vi "Setup.vi"(0 "Power Supply VISA resource name":refnum<visa-resource-name>, 1 "Set Voltage":dbl=3.3 format="%#_13g", 2 "ADC Input Channel 2":tag="cDAQ2Mod3/ai0", 3 "ADC Sample Mode":i32(ring)=10123 items=["Finite Samples"=10178, "Continuous Samples"=10123, "Hardware Timed Single Point"=12522], 4 "Set Max Current for FP":dbl=0.25 format="%#_13g", 5 "Sample Length for ADC mean":i32=100, 6 "ADC Minimum Value":dbl=-10.0 format="%0.2f", 7 "ADC Sampling Rate":dbl=10000.0 format="%0.2f", 8 "ADC Maximum Value":dbl=10.0 format="%0.2f") -> (12 "Sample Length for ADC mean 2":i32=100, 13 "Beginning Time Stamp":timestamp, 14 "DAQ Task Out":refnum<k21>, 15 "DAQ Error Out":errorcluster, 16 "VISA resource name out":refnum<visa-resource-name>, 17 "Power Supply Error Out":errorcluster, 18 "LINX Resource":T1={"IO"=enum."Remote", "Interface"=enum."Serial", "LINX Device Config"={"Interface"=enum."Serial", "COM Port"="COM13", "TCP Configuration"={"IP Address"="", "Port"=0}, "Device Family"=1, "Device ID"=1, "Device Name"="myRIO-1900", "TCP Ref"=refnum, "Channels"={"DI"=[0, 1, 2, 3, 4, 5, 6, 7, 8, 9, 10, 11, 12, 13, 14, 15, 16, 17, 18, 19, 20, 21, 22, 23, 24, 25, 26, 27, 28, 29, 30, 31, 32, 33, 34, 35, 36, 37, 38, 39, 40, 41, 42, 43, 44, 45, 46], "DO"=[0, 1, 2, 3, 4, 5, 6, 7, 8, 9, 10, 11, 12, 13, 14, 15, 16, 17, 18, 19, 20, 21, 22, 23, 24, 25, 26, 27, 28, 29, 30, 31, 32, 33, 34, 35, 36, 37, 38, 39, 40, 41, 42, 43, 44, 45, 46], "AI"=[0, 1, 2, 3, 4, 5, 6, 7, 8, 9, 10, 11], "AO"=[], "PWM"=[3, 5, 6, 9, 10], "QE"=[], "UART"=[0, 1], "I2C 2"=[0], "SPI"=[0], "CAN"=[], "Servo"=[], "AI Ref (V)"=0.0, "AI Resolution (Bits)"=0, "AO Ref (V)"=0.0, "AO Resolution (Bits)"=0}}}, 19 "Arduino Error Out":errorcluster={"status"=FALSE, "code"=1073676294, "source"="VISA Read in LVH-LINX.lvlib:Device.lvlib:Serial Read.vi->LVH-LINX.lvlib:Device.lvlib:Wait For Packet.vi->LVH-LINX.lvlib:Device.lvlib:Send Command.vi->LVH-LINX.lvlib:Device.lvlib:Get DIO Channels.vi->LVH-LINX.lvlib:Device.lvlib:Load Device Config.vi->LVH-LINX.lvlib:Device.lvlib:Initialize Device.vi->LVH-LINX.lvlib:Initialize.vi->Untitled 2"})   [LabVIEW 2018]
uses:
  <vilib>/MakerHub/LINX/Private/Type Defs/LINX Ref.ctl
  <vilib>/MakerHub/LINX/Private/Type Defs/Platform.ctl
  <vilib>/MakerHub/LINX/Private/Type Defs/Interface.ctl
  <vilib>/MakerHub/LINX/Private/Device/Type Defs/LINX Device Config.ctl
  <vilib>/MakerHub/LINX/Private/Device/Type Defs/TCP Config.ctl
  <vilib>/MakerHub/LINX/Private/Device/Type Defs/Channels.ctl
  <vilib>/MakerHub/LINX/Public/Utilities/Open Serial.vi
  <vilib>/DAQmx/create/channels.llb/DAQmx Create Channel (AI-Voltage-Basic).vi
  <vilib>/DAQmx/configure/timing.llb/DAQmx Timing (Sample Clock).vi
  <instrlib>/XP Power PLS600/XP Power PLS600.lvlib
  <vilib>/MakerHub/LINX/LMH-LINX.lvlib
  <vilib>/MakerHub/LINX/Private/Device/Device.lvlib
panel:
  in  "Serial Port for Arduino":refnum<visa-resource-name>="N/A"
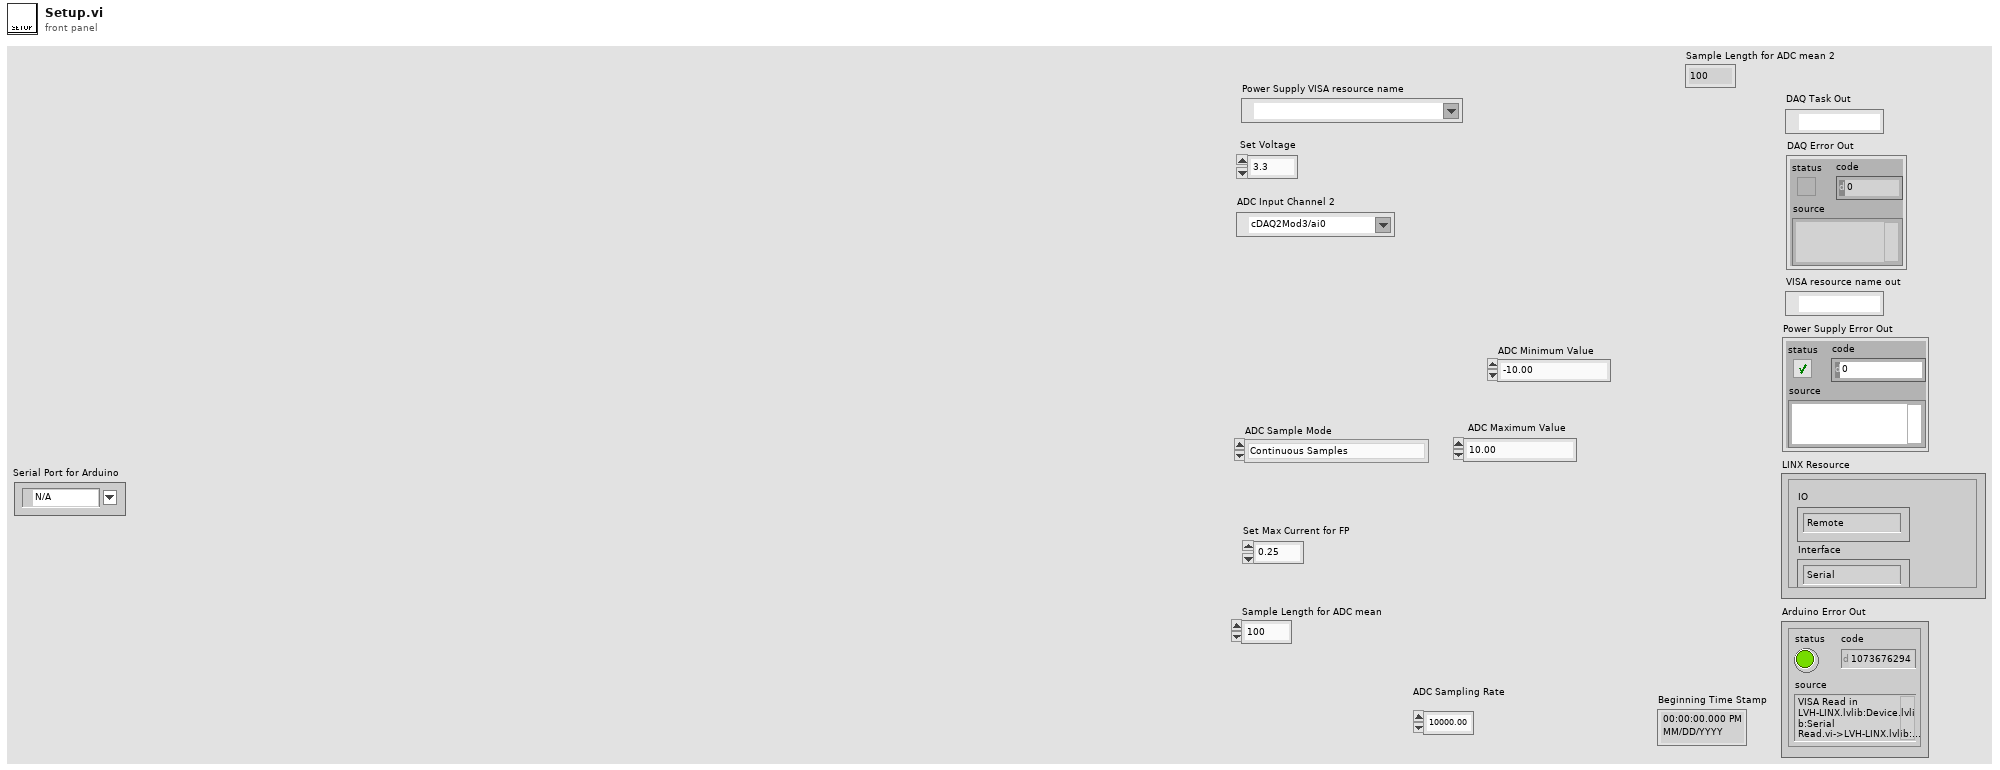
[diagram p1: front panel]
types:
  T1 = typedef "LMH-LINX.lvlib/LINX Ref.ctl" = cluster{"IO":T2, "Interface":T3, "LINX Device Config":T4}
  T2 = typedef "LMH-LINX.lvlib/Platform.ctl" = enum16{"Remote", "Local"}
  T3 = typedef "LMH-LINX.lvlib/Interface.ctl" = enum16{"Serial", "TCP"}
  T4 = typedef "LMH-LINX.lvlib/Device.lvlib/LINX Device Config.ctl" = cluster{"Interface":T3, "COM Port":refnum<visa-resource-name>, "TCP Configuration":T5, "Device Family":u8, "Device ID":u8, "Device Name":string, "TCP Ref":refnum<k5>, "Channels":T6}
  T5 = typedef "LMH-LINX.lvlib/Device.lvlib/TCP Config.ctl" = cluster{"IP Address":string, "Port":u16}
  T6 = typedef "LMH-LINX.lvlib/Channels.ctl" = cluster{"DI":u8[], "DO":u8[], "AI":u8[], "AO":u8[], "PWM":u8[], "QE":u8[], "UART":u8[], "I2C 2":u8[], "SPI":u8[], "CAN":u8[], "Servo":u8[], "AI Ref (V)":dbl, "AI Resolution (Bits)":u8, "AO Ref (V)":dbl, "AO Resolution (Bits)":u8}
  T7 = cluster{"Baud Rate":u32, "Parity":u16, "Data Bits":u16, "Stop Bits":u16, "Flow Control":u16}
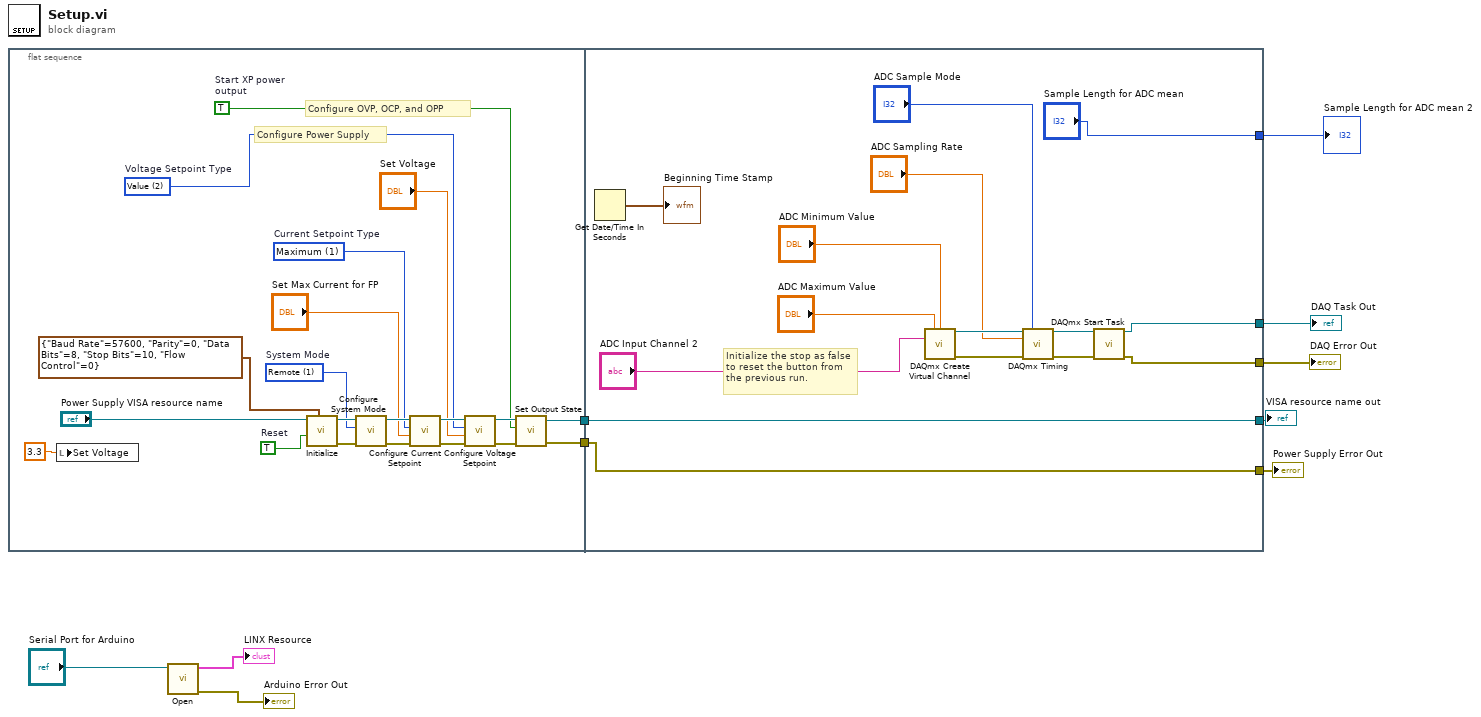
[diagram p0: block diagram]
diagram:
  n1 = flat-sequence {
    tunnel: [w13] -> w10
    tunnel: [w12] -> w9
    tunnel: w10 -> [w35]
    tunnel: w9 -> [w34]
    tunnel: [w35] -> w6
    tunnel: [w34] -> w5
    tunnel: [w33] -> w4
    tunnel: [w32] -> w3
    tunnel: ["Sample Length for ADC mean"] -> w1
    frame #0 {
      w19 = 2 items=["Minimum", "Maximum", "Value"]  # Voltage Setpoint Type
      w17 = TRUE  # Start XP power output
      w18 = 1 items=["Minimum", "Maximum", "Value"]  # Current Setpoint Type
      w16 = 1 items=["Local", "Remote", "Remote with Lock", "Voltage", "Current", "Dual"]  # System Mode
      w14 = TRUE  # Reset
      # "Configure Power Supply"
      # "Configure OVP, OCP, and OPP"
      n2 = local write "Set Voltage"(3.3) -> ()
      n3 = call <instrlib>:"Initialize.vi"("Serial Configuration"=T7 {"Baud Rate"=57600, "Parity"=0, "Data Bits"=8, "Stop Bits"=10, "Flow Control"=0}, "Reset (True)"=w14, "VISA resource name"="Power Supply VISA resource name") -> ("error out"=w20:errorcluster, "VISA resource name out"=w21:refnum<visa-resource-name>)  [unwired: 7 in]
      n4 = call <instrlib>:"Configure System Mode.vi"("error in (no error)"=w20, "System Mode (0: Local)"=w16, "VISA resource name"=w21) -> ("error out"=w30:errorcluster, "VISA resource name out"=w29:refnum<visa-resource-name>)  [unwired: 7 in]
      n5 = call <instrlib>:"Configure Current Setpoint.vi"("error in (no error)"=w30, "Current Setpoint (0 amperes)"="Set Max Current for FP", "Current Setpoint Type (0: Minimum)"=w18, "VISA resource name"=w29) -> ("error out"=w27:errorcluster, "VISA resource name out"=w28:refnum<visa-resource-name>)  [unwired: 6 in]
      n6 = call <instrlib>:"Configure Voltage Setpoint.vi"("error in (no error)"=w27, "Voltage Setpoint (0 volts)"="Set Voltage", "Voltage Setpoint Type (0: Minimum)"=w19, "VISA resource name"=w28) -> ("error out"=w26:errorcluster, "VISA resource name out"=w25:refnum<visa-resource-name>)  [unwired: 6 in]
      n7 = call <instrlib>:"Set Output State.vi"("error in (no error)"=w26, "Output State (F: Disable)"=w17, "VISA resource name"=w25) -> ("error out"=w12:errorcluster, "VISA resource name out"=w13:refnum<visa-resource-name>)  [unwired: 7 in]
    }
    frame #1 {
      # "Initialize the stop as false\nto reset the button from\nthe previous run."
      n8 = Get Date/Time In Seconds() -> (seconds since 1Jan1904=→"Beginning Time Stamp":timestamp)
      n9 = call-poly <vilib>:"DAQmx Create Virtual Channel.vi"("maximum value"="ADC Maximum Value", "minimum value"="ADC Minimum Value", "physical channels"="ADC Input Channel 2") -> ("task out"=w42:refnum<k21>, "error out"=w39:errorcluster)  [unwired: 11 in]
      n10 = call-poly <vilib>:"DAQmx Timing.vi"("task/channels in"=w42, "sample mode"="ADC Sample Mode", "rate"="ADC Sampling Rate", "error in"=w39) -> ("task out"=w41:refnum<k21>, "error out"=w40:errorcluster)  [unwired: 10 in]
      n11 = call <vilib>:"DAQmx Start Task.vi"("task/channels in"=w41, "error in"=w40) -> ("task out"=w32:refnum<k21>, "error out"=w33:errorcluster)  [unwired: 12 in]
    }
  }
  n12 = call-poly <vilib>:"Open.vi"("Serial Port"="Serial Port for Arduino") -> ("Error Out"=→"Arduino Error Out":errorcluster, "LINX Resource"=→"LINX Resource":T1)  [unwired: 8 in, 1 out]
  "VISA resource name out" <- w6
  "Power Supply Error Out" <- w5
  "DAQ Error Out" <- w4
  "DAQ Task Out" <- w3
  "Sample Length for ADC mean 2" <- w1
